vi "StringToArrayStringPC.vi"(8 "sortie d'erreur":errorcluster, 11 "Return value":string) -> (0 "sortie d'erreur":errorcluster, 3 "Data":T1)   [LabVIEW 2020]
uses:
  <vilib>/Utility/error.llb/Error Cluster From Error Code.vi
  <vilib>/ErrorRing/Error Ring.xnode
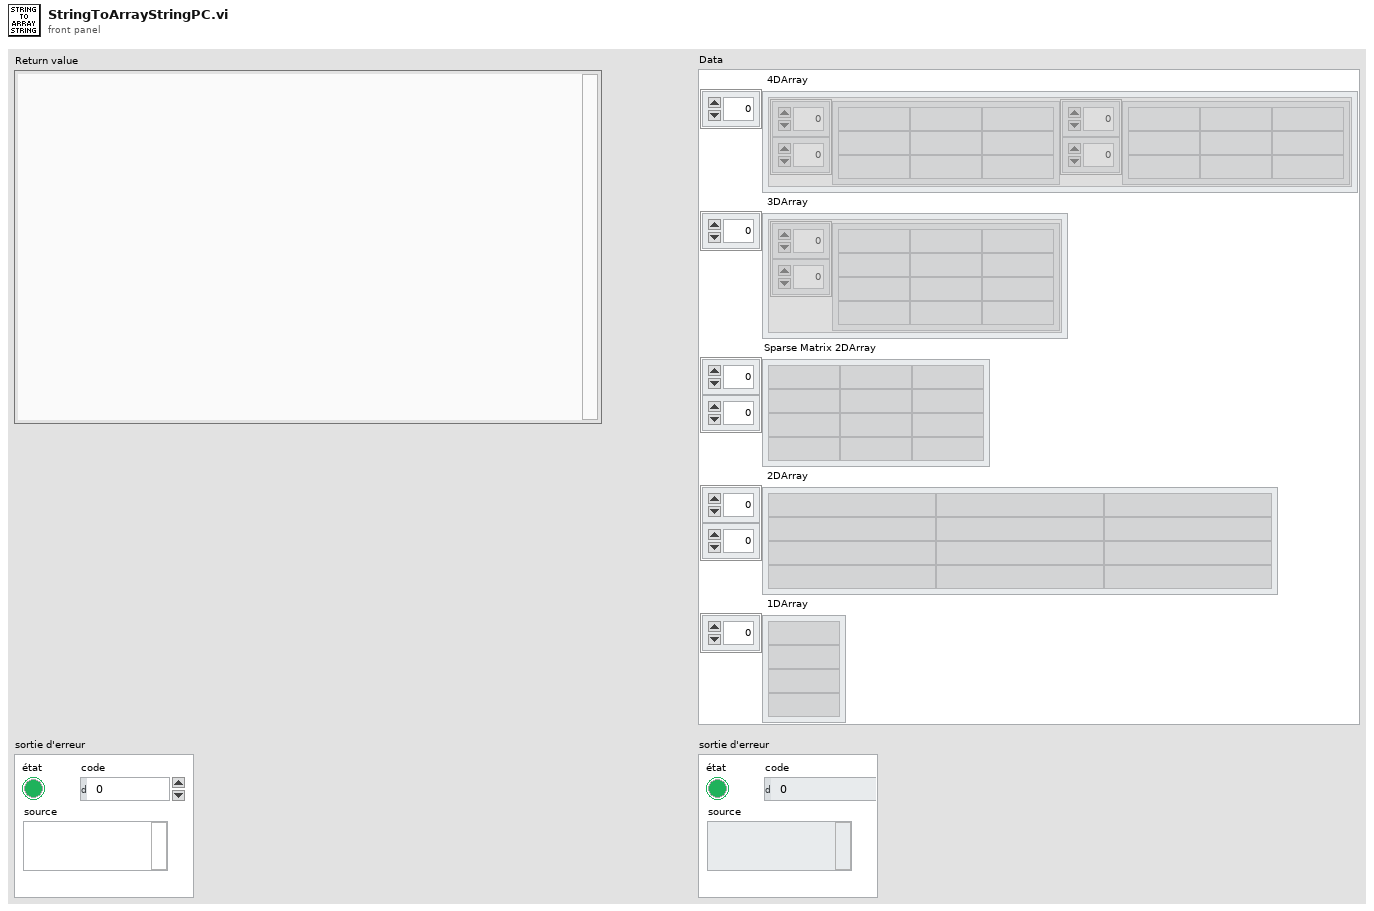
[diagram p1: front panel]
types:
  T1 = cluster{" 4DArray":cluster{"1":string[][], "2":string[][]}[], " 3DArray":cluster{"Tableau":string[][]}[], "Sparse Matrix 2DArray":string[][], " 2DArray":string[][], " 1DArray":string[]}
  T2 = cluster{"String 4DArray":cluster{"1":string[][], "2":string[][]}[], cluster{string[][]}[], string[][], string[][], "string array":string[]}
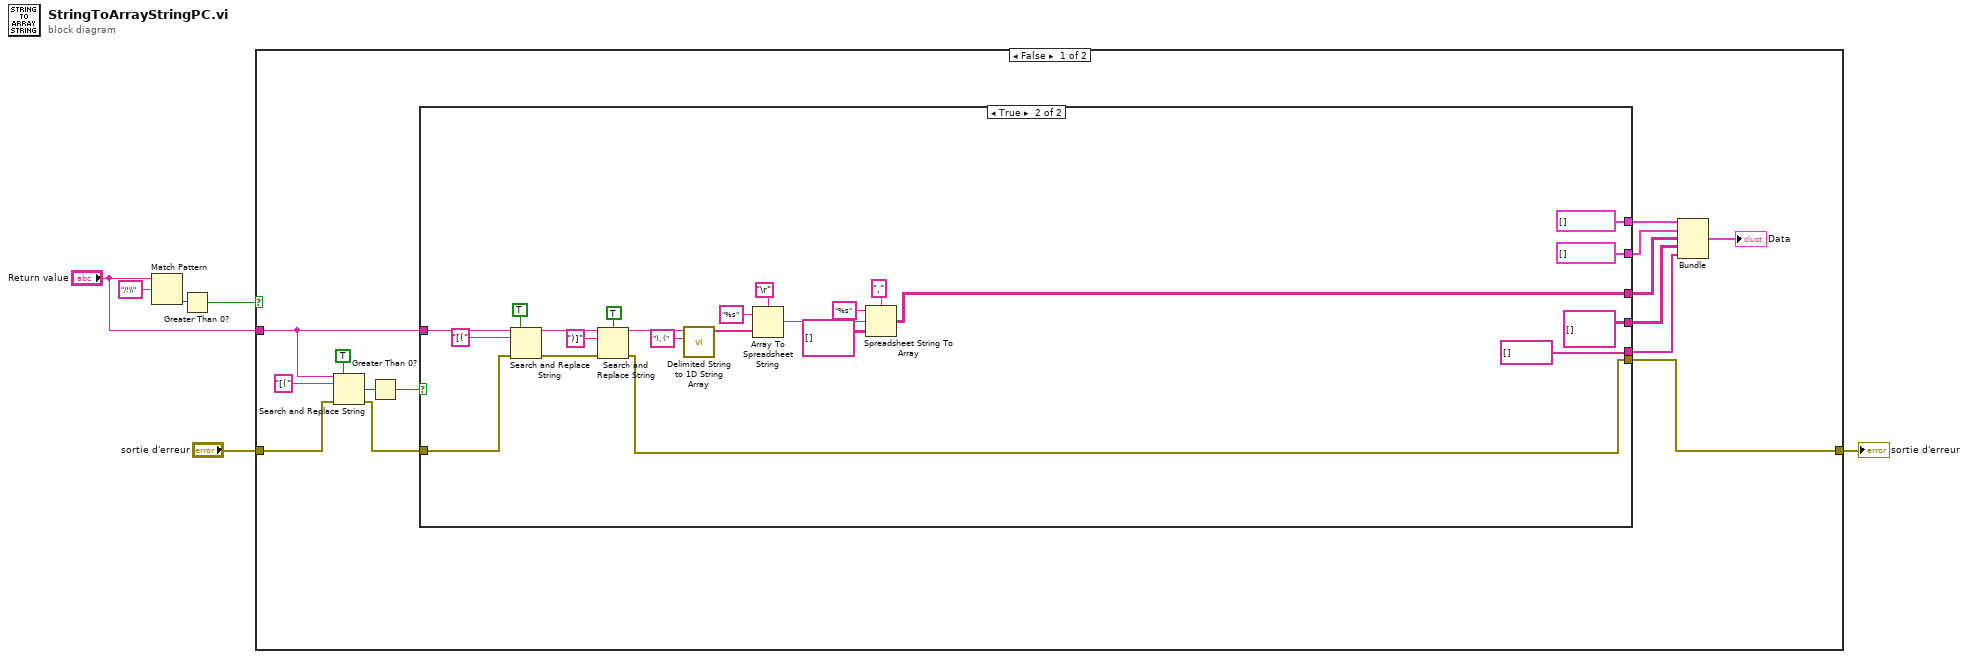
[diagram p0: block diagram]
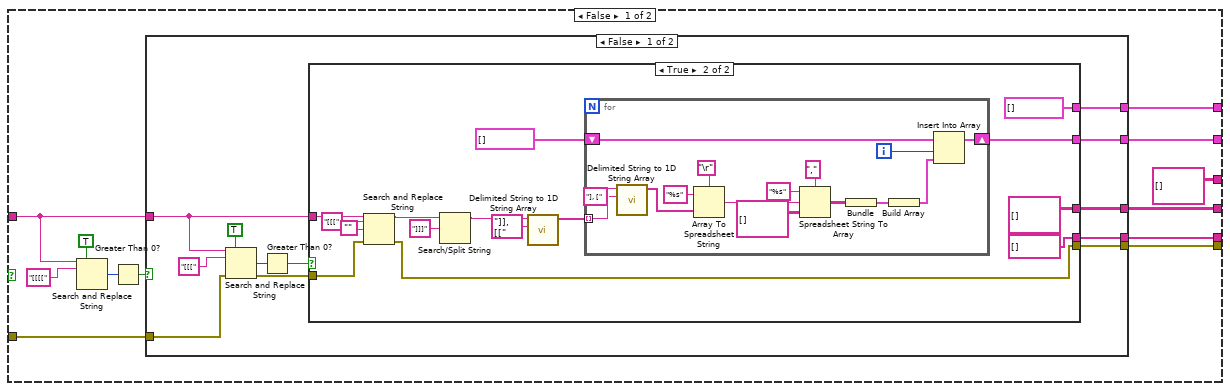
[diagram p2: hidden frame]
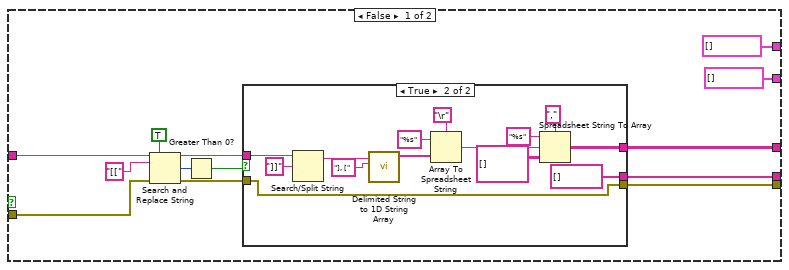
[diagram p3: hidden frame]
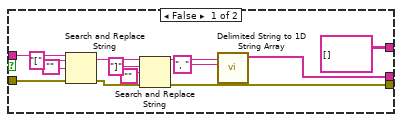
[diagram p4: hidden frame]
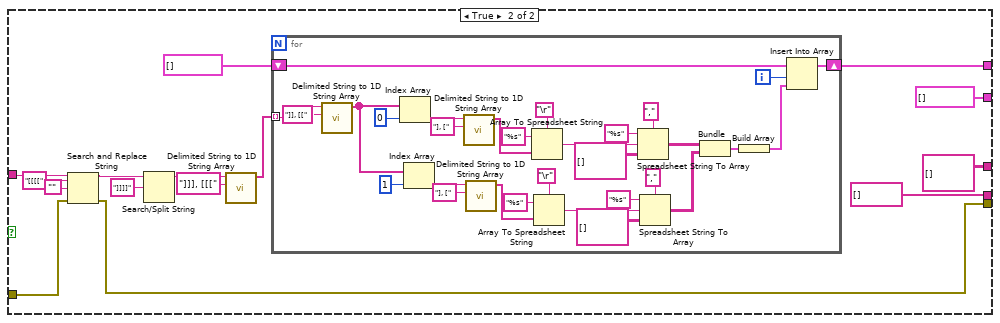
[diagram p5: hidden frame]
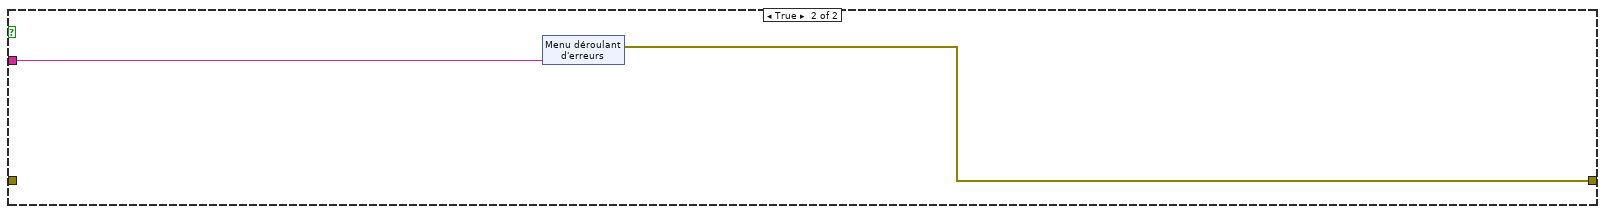
[diagram p6: hidden frame]
diagram:
  n1 = Match Pattern(string="Return value", regular expression="/!\\" ("expression régulière")) -> (offset past match=w5:i32)  [unwired: 1 in, 3 out]
  n2 = Greater Than 0?(x=w5) -> (x > 0?=w1:bool)
  n3 = case shown="False" w1 {
    tunnel: "Return value" -> [w15 w184]
    tunnel: [w20 w183] -> w3
    tunnel: "sortie d'erreur" -> [w14 _]
    frame False {
      n4 = Search and Replace String(replace all?=TRUE ("replace all? (F)"), input string=w15, search string="[(", error in=w14) -> (number of replacements=w18:i32, error out=w13:errorcluster)  [unwired: 4 in, 2 out]
      n5 = Greater Than 0?(x=w18) -> (x > 0?=w16:bool)
      n6 = case shown="True" w16 {
        tunnel: [w32 string[] [] ("string array")] -> w8
        tunnel: [w31 string[][] []] -> w9
        tunnel: [w30 cluster{string[][]}[] []] -> w11
        tunnel: w13 -> [w29 w162]
        tunnel: [w28 w172] -> w20
        tunnel: w15 -> [w24 w163]
        tunnel: [w22 cluster{"1":string[][], "2":string[][]}[] [] ("String 4DArray")] -> w12
        tunnel: [string[][] [] w171] -> w10
        frame False {
          n7 = Search and Replace String(replace all?=TRUE ("replace all? (F)"), input string=w24, search string="[[[[") -> (number of replacements=w26:i32)  [unwired: 5 in, 3 out]
          n8 = Greater Than 0?(x=w26) -> (x > 0?=w23:bool)
          n9 = case shown="False" w23 {
            tunnel: [w40 string[] [] ("string array")] -> w32
            tunnel: [w39 string[][] []] -> w31
            tunnel: [w38 cluster{string[][]}[] []] -> w30
            tunnel: w24 -> [w37 w122]
            tunnel: w29 -> [w36 w121]
            tunnel: [w34 w120] -> w28
            tunnel: [w33 w115] -> w22
            frame False {
              n10 = Search and Replace String(replace all?=TRUE ("replace all? (F)"), input string=w37, search string="[[[", error in=w36) -> (number of replacements=w43:i32, error out=w35:errorcluster)  [unwired: 4 in, 2 out]
              n11 = Greater Than 0?(x=w43) -> (x > 0?=w42:bool)
              n12 = case shown="True" w42 {
                tunnel: w37 -> [w52 w89]
                tunnel: [w51 string[][] []] -> w39
                tunnel: [w50 string[] [] ("string array")] -> w40
                tunnel: [cluster{string[][]}[] [] w92] -> w38
                tunnel: w35 -> [w48 w87]
                tunnel: [w46 w86] -> w34
                tunnel: [cluster{"1":string[][], "2":string[][]}[] [] ("String 4DArray") cluster{"1":string[][], "2":string[][]}[] [] ("String 4DArray")] -> w33
                frame False {
                  n13 = Search and Replace String(replace all?=TRUE ("replace all? (F)"), input string=w52, search string="[[", error in=w48) -> (result string=w53:string, number of replacements=w55:i32, error out=w47:errorcluster)  [unwired: 4 in, 1 out]
                  n14 = Greater Than 0?(x=w55) -> (x > 0?=w54:bool)
                  n15 = case shown="True" w54 {
                    tunnel: w53 -> [w64 w81]
                    tunnel: [string[][] [] w73] -> w51
                    tunnel: [w62 string[] [] ("string array")] -> w50
                    tunnel: w47 -> [w60 w71]
                    tunnel: [w58 w71] -> w46
                    frame False {
                      n16 = Search and Replace String(input string=w64, search string="[", replace string="", error in=w60) -> (result string=w65:string, error out=w59:errorcluster)  [unwired: 4 in, 2 out]
                      n17 = Search and Replace String(input string=w65, search string="]", replace string="", error in=w59) -> (result string=w63:string, error out=w58:errorcluster)  [unwired: 4 in, 2 out]
                      n18 = call <vilib>:"Delimited String to 1D String Array.vi"("delimiter"=", ", "delimited string"=w63) -> ("string array"=w62:string[])  [unwired: 9 in]
                    }
                    frame True {
                      n19 = Search/Split String(string=w81, search string/char (-)="]]" ("chaîne/car. recherché (-)")) -> (substring before match=w80:string)  [unwired: 1 in, 2 out]
                      n20 = call <vilib>:"Delimited String to 1D String Array.vi"("delimiter"="], [", "delimited string"=w80) -> ("string array"=w83:string[])  [unwired: 9 in]
                      n21 = Array To Spreadsheet String(delimiter (Tab)="\r", array=w83, 3:"%s" ("chaîne de format")) -> (spreadsheet string=w74:string)
                      n22 = Spreadsheet String To Array(delimiter (Tab)="," ("séparateur (Tabulation)"), format string="%s" ("chaîne de format"), spreadsheet string=w74, array type (2D Dbl)=string[][] []) -> (array=w73:string[][])
                    }
                  }
                }
                frame True {
                  n23 = Search and Replace String(input string=w89, search string="[[[", replace string="", error in=w87) -> (result string=w88:string, error out=w86:errorcluster)  [unwired: 4 in, 2 out]
                  n24 = Search/Split String(string=w88, search string/char (-)="]]]" ("chaîne/car. recherché (-)")) -> (substring before match=w93:string)  [unwired: 1 in, 2 out]
                  n25 = call <vilib>:"Delimited String to 1D String Array.vi"("delimiter"="]], [[", "delimited string"=w93) -> ("string array"=w96:string[])  [unwired: 9 in]
                  n26 = for {
                    tunnel: w96 -> [w111] mode=indexing
                    shift-right: [w100] -> w92
                    shift-left: cluster{string[][]}[] [] -> [w101]
                    i -> [w102]
                    n27 = call <vilib>:"Delimited String to 1D String Array.vi"("delimiter"="], [", "delimited string"=w111) -> ("string array"=w107:string[])  [unwired: 9 in]
                    n28 = Array To Spreadsheet String(delimiter (Tab)="\r", array=w107, 3:"%s" ("chaîne de format")) -> (spreadsheet string=w106:string)
                    n29 = Spreadsheet String To Array(delimiter (Tab)="," ("séparateur (Tabulation)"), format string="%s" ("chaîne de format"), spreadsheet string=w106, array type (2D Dbl)=string[][] []) -> (array=w105:string[][])
                    n30 = Bundle(w105) -> (w104:cluster{string[][]})  [unwired: 1 in]
                    n31 = Build Array(w104) -> (w103:cluster{string[][]}[])
                    n32 = Insert Into Array(array=w101, index=w102, new element=w103) -> (w100:cluster{string[][]}[])
                  }
                }
              }
            }
            frame True {
              n33 = Search and Replace String(input string=w122, search string="[[[[", replace string="", error in=w121) -> (result string=w123:string, error out=w120:errorcluster)  [unwired: 4 in, 2 out]
              n34 = Search/Split String(string=w123, search string/char (-)="]]]]" ("chaîne/car. recherché (-)")) -> (substring before match=w118:string)  [unwired: 1 in, 2 out]
              n35 = call <vilib>:"Delimited String to 1D String Array.vi"("delimiter"="]]], [[[", "delimited string"=w118) -> ("string array"=w116:string[])  [unwired: 9 in]
              n36 = for {
                tunnel: w116 -> [w159] mode=indexing
                shift-right: [w155] -> w115
                shift-left: cluster{"1":string[][], "2":string[][]}[] [] ("String 4DArray") -> [w156]
                i -> [w157]
                n37 = call <vilib>:"Delimited String to 1D String Array.vi"("delimiter"="]], [[", "delimited string"=w159) -> ("string array"=w134:string[])  [unwired: 9 in]
                n38 = Index Array(array=w134, index=0 ("indice")) -> (element=w143:string)
                n39 = Index Array(array=w134, index=1 ("indice")) -> (element=w132:string)
                n40 = call <vilib>:"Delimited String to 1D String Array.vi"("delimiter"="], [", "delimited string"=w143) -> ("string array"=w146:string[])  [unwired: 9 in]
                n41 = call <vilib>:"Delimited String to 1D String Array.vi"("delimiter"="], [", "delimited string"=w132) -> ("string array"=w135:string[])  [unwired: 9 in]
                n42 = Array To Spreadsheet String(delimiter (Tab)="\r", array=w146, 3:"%s" ("chaîne de format")) -> (spreadsheet string=w147:string)
                n43 = Array To Spreadsheet String(delimiter (Tab)="\r", array=w135, 3:"%s" ("chaîne de format")) -> (spreadsheet string=w136:string)
                n44 = Spreadsheet String To Array(delimiter (Tab)="," ("séparateur (Tabulation)"), format string="%s" ("chaîne de format"), spreadsheet string=w147, array type (2D Dbl)=string[][] []) -> (array=w145:string[][])
                n45 = Spreadsheet String To Array(delimiter (Tab)="," ("séparateur (Tabulation)"), format string="%s" ("chaîne de format"), spreadsheet string=w136, array type (2D Dbl)=string[][] []) -> (array=w131:string[][])
                n46 = Bundle(w145, w131) -> (w154:cluster{string[][], string[][]})  [unwired: 1 in]
                n47 = Build Array(w154) -> (w130:cluster{string[][], string[][]}[])
                n48 = Insert Into Array(array=w156, index=w157, new element=w130) -> (w155:cluster{"1":string[][], "2":string[][]}[])
              }
            }
          }
        }
        frame True {
          n49 = Search and Replace String(replace all?=TRUE ("replace all? (F)"), input string=w163, search string="[(", error in=w162) -> (result string=w160:string, error out=w161:errorcluster)  [unwired: 4 in, 2 out]
          n50 = Search and Replace String(case sensitive?=TRUE ("ignorer la casse ? (F)"), input string=w160, search string=")]" ("chaîne recherchée"), error in=w161) -> (result string=w181:string, error out=w172:errorcluster)  [unwired: 4 in, 2 out]
          n51 = call <vilib>:"Delimited String to 1D String Array.vi"("delimiter"="), (", "delimited string"=w181) -> ("string array"=w174:string[])  [unwired: 9 in]
          n52 = Array To Spreadsheet String(delimiter (Tab)="\r", array=w174, 3:"%s" ("chaîne de format")) -> (spreadsheet string=w173:string)
          n53 = Spreadsheet String To Array(delimiter (Tab)="," ("séparateur (Tabulation)"), format string="%s" ("chaîne de format"), spreadsheet string=w173, array type (2D Dbl)=string[][] []) -> (array=w171:string[][])
        }
      }
      n54 = Bundle("String 4DArray"=w12, w11, w10, w9, "string array"=w8) -> (→"Data":T2)  [unwired: 1 in]
    }
    frame True {
      n55 = xnode "Menu déroulant d'erreurs"("parameter 0"=w184) -> ("error out"=w183:errorcluster)
    }
  }
  "sortie d'erreur" <- w3
